vi "HTVacuumGUI.CalcDIStatus.vi"(1 "DIStatus":i16, 6 "Color2":u32(colorbox)=16711680, 7 "Color3":u32(colorbox), 8 "Color1":u32(colorbox)=6618880, 9 "Color Control Ref":refnum<vi>, 11 "Boolen Ref":refnum<vi>) -> ()   [LabVIEW 2014, in "HTVacuumGUI.lvlib"]
uses:
  HTVacuumGUI.lvlib
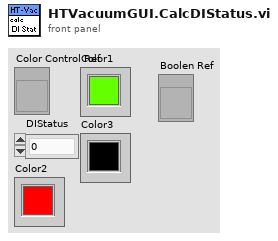
[diagram p1: front panel]
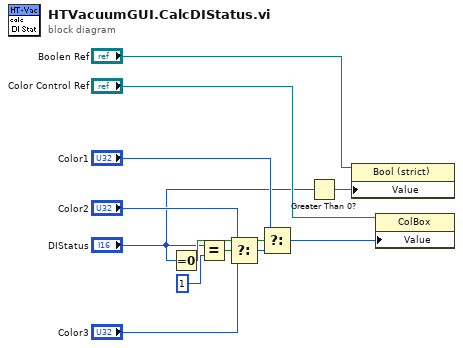
[diagram p0: block diagram]
diagram:
  n1 = Equal To 0?(x="DIStatus") -> (x = 0?=w9:bool)
  n2 = Equal?(x="DIStatus", y=u32 1) -> (x = y?=w11:bool)
  n3 = Select(t="Color2", s=w11, f="Color3") -> (s? t:f=w12:u32)
  n4 = Select(t="Color1", s=w9, f=w12) -> (s? t:f=w4:u32)
  n5 = Greater Than 0?(x="DIStatus") -> (x > 0?=w1:bool)
  n6 = property class="Bool (strict)"(reference="Boolen Ref", "Value"=w1) -> ()  [unwired: 1 in, 2 out]
  n7 = property class="ColBox"(reference="Color Control Ref", "Value"=w4) -> ()  [unwired: 1 in, 2 out]
